vi "ElevatorGetPosition.vi"() -> (1 "ElevOuterHeight":dbl, 3 "ElevStage3Height":dbl)   [LabVIEW 2023]
doc: "Reads the Elevator's actual measured height from the Elevator Global ElevatorPositionHeight\n\nOutputs:\n--ElevHeight--numeric--inches"
uses:
  ElevatorGlobal.vi
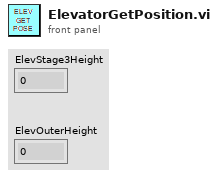
[diagram p1: front panel]
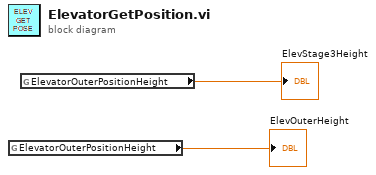
[diagram p0: block diagram]
diagram:
  n1 = global read "ElevatorGlobal.vi" "ElevatorOuterPositionHeight"() -> (→"ElevOuterHeight":dbl)
  n2 = global read "ElevatorGlobal.vi" "ElevatorOuterPositionHeight"() -> (→"ElevStage3Height":dbl)
